vi "Grad_Adapt.vi"(4 "Gamma":T1, 5 "phi_du":T1, 6 "N":i32, 7 "z":dbl, 8 "error in (no error)":errorcluster, 9 "th_min":T1, 10 "th":T1, 11 "th_max":T1) -> (0 "error out":errorcluster, 3 "theta_dot":T1)   [LabVIEW 2021]
uses:
  <vilib>/Analysis/Matrix/Datatypes/RealMatrix.ctl
  <vilib>/Analysis/Matrix/Numeric/Multiply/Multiply - RM,RM.vi
  <vilib>/Analysis/Matrix/Numeric/Multiply/Multiply - RM,R.vi
  <vilib>/Analysis/Matrix/NI_Matrix.lvlib
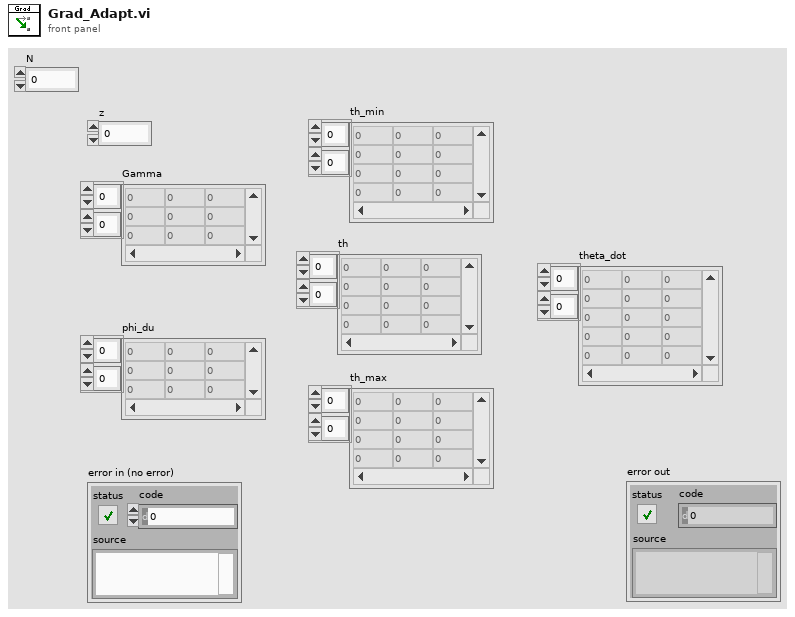
[diagram p1: front panel]
types:
  T1 = typedef "NI_Matrix.lvlib/RealMatrix.ctl" = dbl[][]
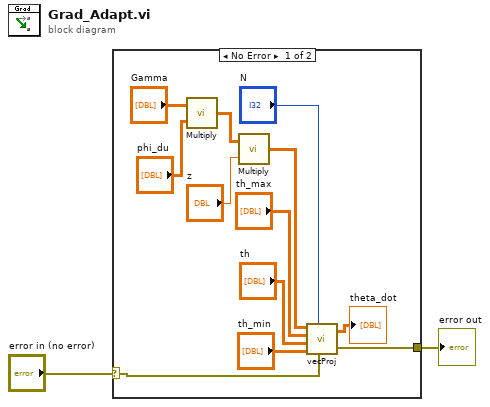
[diagram p0: block diagram]
diagram:
  n1 = case shown="No Error" "error in (no error)" {
    selector: "error in (no error)" -> [w4 w15]
    tunnel: [w3 w15] -> w1
    frame No Error {
      n2 = call-poly <vilib>:"Multiply.vi"("Real Matrix B"="phi_du", "Real Matrix A"="Gamma") -> ("A * B"=w12:T1)
      n3 = call-poly <vilib>:"Multiply.vi"("Real Scalar c"="z", "Real Matrix A"=w12) -> ("A * c"=w7:T1)
      n4 = call "vecProj.vi"("error in (no error)"=w4, "N"="N", "th_min"="th_min", "th"="th", "th_max"="th_max", "a"=w7) -> ("error out"=w3:errorcluster, "Proj_th (a)"=→"theta_dot":T1)
    }
    frame Error {
    }
  }
  "error out" <- w1
